vi "Test MQTT-3.1.3-5.vi"(8 "error in (no error)":errorcluster) -> (0 "error out":errorcluster)   [LabVIEW 2013]
uses:
  <vilib>/LabVIEW Open Source Project/MQTT Control Packets/Control Packets/CONNACK/Connect Return Code -- enum.ctl
  <vilib>/addons/_JKI Toolkits/Caraya/classes/Test/Test.lvclass
  <vilib>/LabVIEW Open Source Project/MQTT Control Packets/Control Packets/CONNACK/CONNACK.lvclass
  <vilib>/addons/_JKI Toolkits/Caraya/classes/Assert/Assert.lvclass
  <vilib>/LabVIEW Open Source Project/MQTT Client/Client class/Client.lvclass
  <vilib>/LabVIEW Open Source Project/MQTT Connection/MQTT_Base/Base Class/MQTT_Base.lvclass
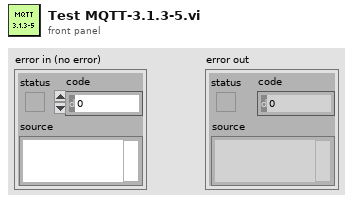
[diagram p1: front panel]
types:
  T1 = typedef "MQTT_Control_Packets.lvlib/CONNACK.lvclass/Connect Return Code -- enum.ctl" = enum16{"Connection accepted", "Unacceptable protocol version", "Identifier Rejected", "Server Unavailable", "Bad Username or Password", "Not Authorized"}
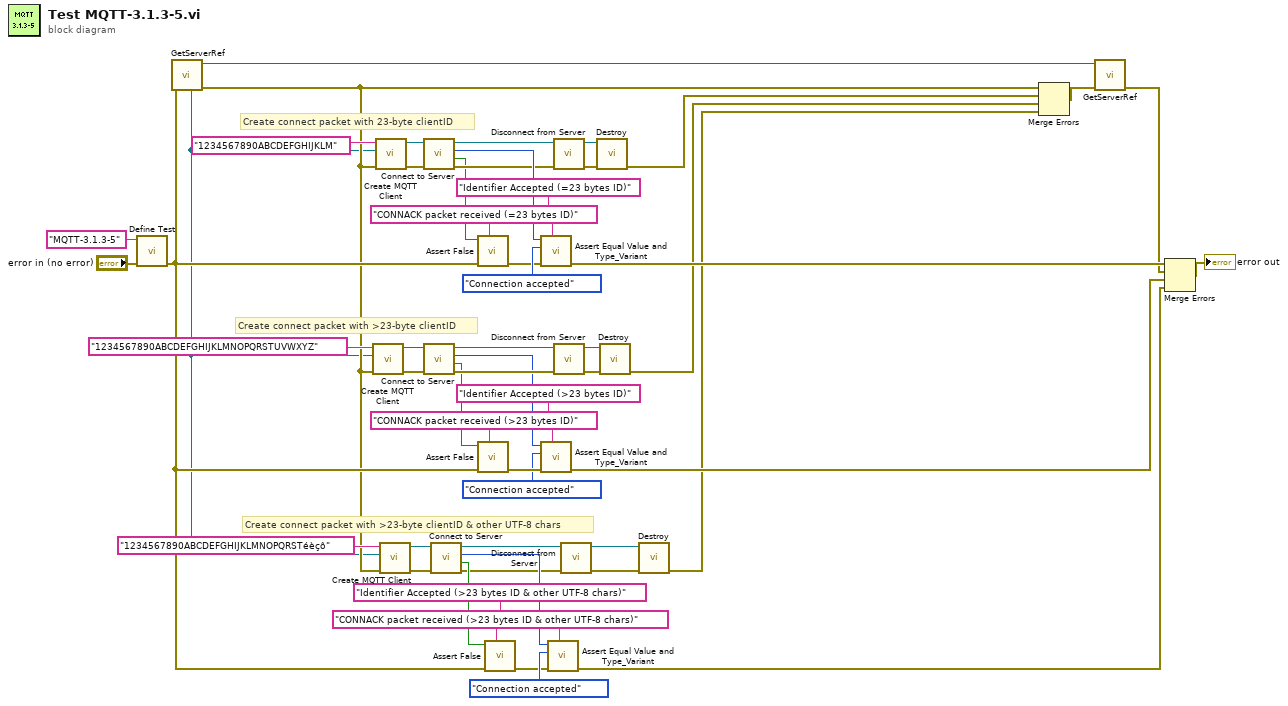
[diagram p0: block diagram]
diagram:
  # "Create connect packet with >23-byte clientID & other UTF-8 chars"
  # "Create connect packet with >23-byte clientID"
  # "Create connect packet with 23-byte clientID"
  n1 = call <vilib>:"Define Test.vi"("error in (no error)"="error in (no error)", "Label (VI Title)"="MQTT-3.1.3-5") -> ("error out"=w14:errorcluster)  [unwired: 9 in]
  n2 = call "GetServerRef.vi"("error in"=w14) -> ("error out"=w12:errorcluster, "Created"=w46:bool, "Connection Config"=w1:refnum<class "Connection.lvclass">)  [unwired: 6 in, 2 out]
  n3 = call <vilib>:"Create MQTT Client.vi"("error in (no error)"=w12, "Connection Configuration"=w1, "ID (empty:generate new)"="1234567890ABCDEFGHIJKLMNOPQRSTUVWXYZ" ("Client ID (empty: generate new)")) -> ("error out"=w34:errorcluster, "Client out"=w33:refnum<class "Client.lvclass">)  [unwired: 7 in]
  n4 = call <vilib>:"Create MQTT Client.vi"("error in (no error)"=w12, "Connection Configuration"=w1, "ID (empty:generate new)"="1234567890ABCDEFGHIJKLM" ("Client ID (empty: generate new)")) -> ("error out"=w41:errorcluster, "Client out"=w42:refnum<class "Client.lvclass">)  [unwired: 7 in]
  n5 = call <vilib>:"Create MQTT Client.vi"("error in (no error)"=w12, "Connection Configuration"=w1, "ID (empty:generate new)"="1234567890ABCDEFGHIJKLMNOPQRSTéèçô" ("Client ID (empty: generate new)")) -> ("error out"=w17:errorcluster, "Client out"=w18:refnum<class "Client.lvclass">)  [unwired: 7 in]
  n6 = call <vilib>:"Connect to Server.vi"("error in (no error)"=w41, "Client in"=w42) -> ("error out"=w38:errorcluster, "timed out"=w37:bool, "Return Code"=w40:T1, "Client out"=w39:refnum<class "Client.lvclass">)  [unwired: 6 in]
  n7 = call <vilib>:"Connect to Server.vi"("error in (no error)"=w34, "Client in"=w33) -> ("error out"=w36:errorcluster, "timed out"=w25:bool, "Return Code"=w26:T1, "Client out"=w35:refnum<class "Client.lvclass">)  [unwired: 6 in]
  n8 = call <vilib>:"Connect to Server.vi"("error in (no error)"=w17, "Client in"=w18) -> ("error out"=w15:errorcluster, "timed out"=w24:bool, "Return Code"=w23:T1, "Client out"=w16:refnum<class "Client.lvclass">)  [unwired: 6 in]
  n9 = call <vilib>:"Assert False.vi"("Label"="CONNACK packet received (=23 bytes ID)", "error in (no error)"=w14, "False?"=w37) -> ("error out"=w48:errorcluster)  [unwired: 8 in]
  n10 = call <vilib>:"Assert False.vi"("Label"="CONNACK packet received (>23 bytes ID)", "error in (no error)"=w14, "False?"=w25) -> ("error out"=w30:errorcluster)  [unwired: 8 in]
  n11 = call <vilib>:"Assert False.vi"("Label"="CONNACK packet received (>23 bytes ID & other UTF-8 chars)", "error in (no error)"=w14, "False?"=w24) -> ("error out"=w20:errorcluster)  [unwired: 8 in]
  n12 = call <vilib>:"Assert Equal Value and Type_Variant.vi"("Label"="Identifier Accepted (=23 bytes ID)", "error in (no error)"=w48, "Y"=Connect_Return_Code_--_enum."Connection accepted" ("Return Code"), "X"=w40) -> ("error out"=w53:errorcluster)  [unwired: 7 in]
  n13 = call <vilib>:"Assert Equal Value and Type_Variant.vi"("Label"="Identifier Accepted (>23 bytes ID)", "error in (no error)"=w30, "Y"=Connect_Return_Code_--_enum."Connection accepted" ("Return Code"), "X"=w26) -> ("error out"=w27:errorcluster)  [unwired: 7 in]
  n14 = call <vilib>:"Assert Equal Value and Type_Variant.vi"("Label"="Identifier Accepted (>23 bytes ID & other UTF-8 chars)", "error in (no error)"=w20, "Y"=Connect_Return_Code_--_enum."Connection accepted" ("Return Code"), "X"=w23) -> ("error out"=w11:errorcluster)  [unwired: 7 in]
  n15 = call <vilib>:"Disconnect from Server.vi"("error in (no error)"=w38, "Client in"=w39) -> ("error out"=w4:errorcluster, "Client out"=w2:refnum<class "Client.lvclass">)  [unwired: 7 in, 1 out]
  n16 = call <vilib>:"Disconnect from Server.vi"("error in (no error)"=w36, "Client in"=w35) -> ("error out"=w6:errorcluster, "Client out"=w7:refnum<class "Client.lvclass">)  [unwired: 7 in, 1 out]
  n17 = call <vilib>:"Disconnect from Server.vi"("error in (no error)"=w15, "Client in"=w16) -> ("error out"=w9:errorcluster, "Client out"=w10:refnum<class "Client.lvclass">)  [unwired: 7 in, 1 out]
  n18 = call <vilib>:"Destroy.vi"("error in (no error)"=w4, "MQTT_Base in"=w2) -> ("error out"=w3:errorcluster)  [unwired: 8 in, 1 out]
  n19 = call <vilib>:"Destroy.vi"("error in (no error)"=w6, "MQTT_Base in"=w7) -> ("error out"=w5:errorcluster)  [unwired: 8 in, 1 out]
  n20 = call <vilib>:"Destroy.vi"("error in (no error)"=w9, "MQTT_Base in"=w10) -> ("error out"=w8:errorcluster)  [unwired: 8 in, 1 out]
  n21 = Merge Errors(w12, w3, w5, w8) -> (w45:errorcluster)
  n22 = call "GetServerRef.vi"("error in"=w45, "Destroy (F)"=w46) -> ("error out"=w44:errorcluster)  [unwired: 5 in, 4 out]
  n23 = Merge Errors(w53, w44, w27, w11) -> (→"error out":errorcluster)
